vi "继保开入转.vi"(1 "开入":bool[](array[boolean])=[FALSE, FALSE, FALSE, FALSE, FALSE, FALSE, FALSE, FALSE, FALSE, FALSE, FALSE, FALSE, FALSE, FALSE, FALSE] caption="开入in") -> (0 "开入out":T1)   [LabVIEW 2015]
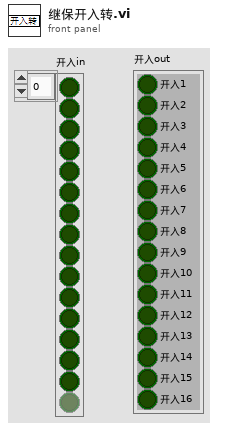
[diagram p1: front panel]
types:
  T1 = cluster{"开入1":bool, "开入2":bool, "开入3":bool, "开入4":bool, "开入5":bool, "开入6":bool, "开入7":bool, "开入8":bool, "开入9":bool, "开入10":bool, "开入11":bool, "开入12":bool, "开入13":bool, "开入14":bool, "开入15":bool, "开入16":bool}
  T2 = cluster{"Boolean":bool, "Boolean":bool, "Boolean":bool, "Boolean":bool, "Boolean":bool, "Boolean":bool, "Boolean":bool, "Boolean":bool, "Boolean":bool, "Boolean":bool, "Boolean":bool, "Boolean":bool, "Boolean":bool, "Boolean":bool, "Boolean":bool, "Boolean":bool}
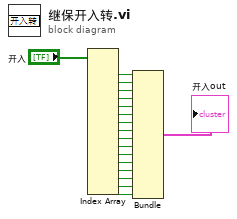
[diagram p0: block diagram]
diagram:
  n1 = Index Array(array="开入") -> (element #1=w17:bool, element #2=w16:bool, element #3=w15:bool, element #4=w14:bool, element #5=w13:bool, element #6=w12:bool, element #7=w11:bool, element #8=w10:bool, element #9=w9:bool, element #10=w8:bool, element #11=w7:bool, element #12=w6:bool, element #13=w4:bool, element #14=w3:bool, element #15=w2:bool, element #16=w1:bool)  [unwired: 16 in]
  n2 = Bundle("Boolean"=w17, "Boolean"=w16, "Boolean"=w15, "Boolean"=w14, "Boolean"=w13, "Boolean"=w12, "Boolean"=w11, "Boolean"=w10, "Boolean"=w9, "Boolean"=w8, "Boolean"=w7, "Boolean"=w6, "Boolean"=w4, "Boolean"=w3, "Boolean"=w2, "Boolean"=w1) -> (→"开入out":T2)  [unwired: 1 in]
